vi "Initialize Core.vi"(8 "error in":errorcluster, 10 "Shared Resources":refnum<class "Shared Resources.lvclass">, 11 "Tx Scheduled Labels Execution Unit in":refnum<class "Tx Scheduled Labels Execution Unit.lvclass">) -> (0 "error out":errorcluster, 3 "Tx Scheduled Labels Execution Unit out":refnum<class "Tx Scheduled Labels Execution Unit.lvclass">)   [LabVIEW 2020, in "AIM ARINC 429 Engine.lvlib" / "Implementation.lvlib" / "Tx Scheduled Labels Execution Unit.lvclass"]
uses:
  Tx Scheduled Labels Execution Unit.lvclass
  Hardware API/AIM ARINC 429 Hardware API.lvlib
  Shared Resources/Shared Resources.lvclass
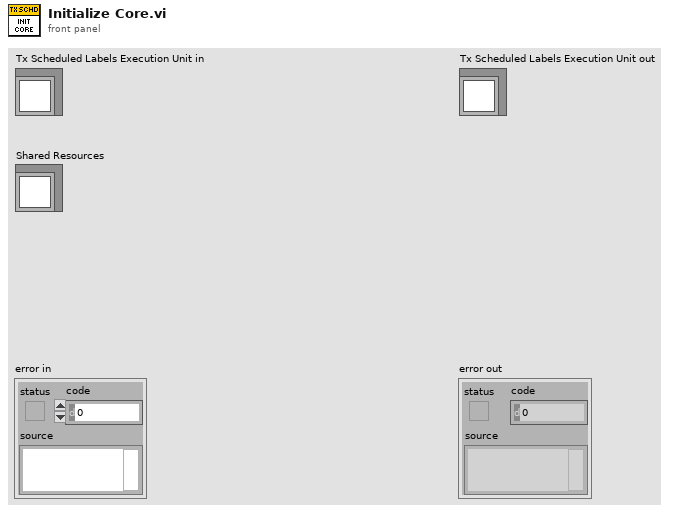
[diagram p1: front panel]
types:
  T1 = typedef "RT Hardware Channel Settings.ctl" = cluster{"channel #":u16, "channel handle":u64, "labels settings for RT":T2[], "speed":T10}
  T2 = typedef "RT Label Settings.ctl" = cluster{"Name":string, "xmlName":string, "label":T3, "transfer period":u32, "SDI_Enabled":bool, "SDI":u8, "parameter driver data":T4, "transfer type":T8, "has timestamp?":bool, "Label Disable/Trigger Channel Reference":T7, "Message Handle":u64, "Initialized?":bool, "Word Initial Raw Value":u32, "Label Timestamp Channel Data Reference":T9, "disabled":bool, "modified":bool}
  T3 = typedef "Label.ctl" = u8
  T4 = typedef "RT Parameters.ctl" = cluster{"parameter definitions":T5[], "Tx parameter refs":T7[]}
  T5 = typedef "Parameter Definition.ctl" = cluster{"start index":i32, "size":i32, "encoding":T6, "signed":bool, "scale multiplier":dbl, "scale offset":dbl, "default value":dbl}
  T6 = typedef "Encoding and Decoding.lvlib/Encoding.ctl" = enum16{"BNR", "BCD", "Discrete"}
  T7 = typedef "Custom Device API.lvlib/Custom Device Item Ref.ctl" = u64
  T8 = typedef "Transfer Type.ctl" = enum16{"Scheduled", "Acyclic", "Block", "Strobe"}
  T9 = typedef "Custom Device API.lvlib/Data Reference.ctl" = i32
  T10 = typedef "Transfer Speed.ctl" = enum16{"LO (12.5 kb/s)", "HI (100 kb/s)"}
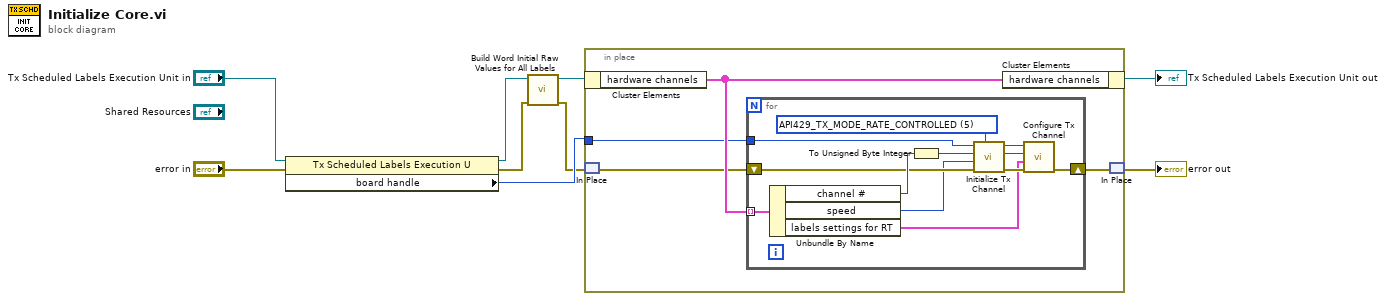
[diagram p0: block diagram]
diagram:
  n1 = property class="Tx Scheduled Labels Execution U"(reference="Tx Scheduled Labels Execution Unit in", error in="error in") -> (reference out=w4:refnum<class "Tx Scheduled Labels Execution Unit.lvclass">, error out=w2:errorcluster, "board handle"=w9:u8)
  n2 = call "Build Word Initial Raw Values for All Labels.vi"("error in"=w2, "Tx Scheduled Labels Execution Unit in"=w4) -> ("error out"=w1:errorcluster, "Tx Scheduled Labels Execution Unit out"=w3:refnum<class "Tx Scheduled Labels Execution Unit.lvclass">)  [unwired: 8 in]
  n3 = in-place {
    in-place-border: w9 -> [w10]
    n4 = in-place-cluster #1(w3) -> ("hardware channels"=w13:T1[])
    n5 = in-place-match #2(w1) -> (w12:errorcluster)
    n6 = for {
      tunnel: w13 -> [w25] mode=indexing
      shift-right: [w16] -> w11
      shift-left: w12 -> [w23]
      tunnel: w10 -> [w22]
      w20 = u32 5 items=["API429_TX_MODE_FRAMING", "API429_TX_MODE_LOOP", "API429_TX_MODE_PHYS_REPLAY", "API429_TX_MODE_FRAMING_DYNTAG", "API429_TX_MODE_FIFO", "API429_TX_MODE_RATE_CONTROLLED"] ("mode")
      n7 = Unbundle By Name(w25) -> ("channel #"=w24:u16, "speed"=w15:T10, "labels settings for RT"=w14:T2[])
      n8 = To Unsigned Byte Integer(number=w24) -> (unsigned 8bit integer=w21:u8)
      n9 = call "Initialize Tx Channel.vi"("mode"=w20, "error in"=w23, "channel speed"=w15, "channel number"=w21, "board handle"=w22) -> ("error out"=w19:errorcluster, "channel number out"=w18:u8, "board handle out"=w17:u8)  [unwired: 4 in]
      n10 = call "Configure Tx Channel.vi"("error in"=w19, "labels settings for RT"=w14, "channel number in"=w18, "board handle in"=w17) -> ("error out"=w16:errorcluster)  [unwired: 4 in, 3 out]
    }
    n11 = in-place-cluster #1("hardware channels"=w13) -> (→"Tx Scheduled Labels Execution Unit out":refnum<class "Tx Scheduled Labels Execution Unit.lvclass">)
    n12 = in-place-match #2(w11) -> (→"error out":errorcluster)
  }
